vi "例4.20-2求方程的根（公式节点）.vi"() -> ()   [LabVIEW 2017]
panel:
  out "x2":dbl
  out "x1":dbl
  in  "c":dbl
  in  "b":dbl
  in  "a":dbl
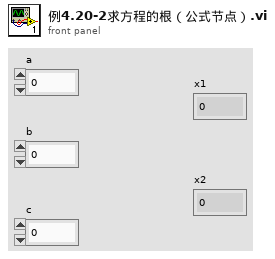
[diagram p1: front panel]
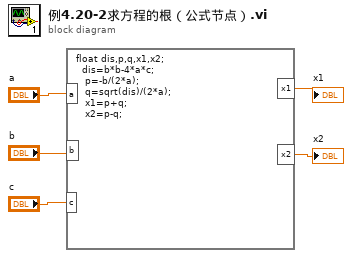
[diagram p0: block diagram]
diagram:
  n1 = formula code="float dis,p,q,x1,x2; \n  dis=b*b-4*a*c;\n   p=-b/(2*a);\n   q=sqrt(dis)/(2*a);\n   x1=p+q;\n   x2=p-q;"("a"="a", "b"="b", "c"="c") -> ("x1"=→"x1":dbl, "x2"=→"x2":dbl)
